vi "Producto extraccion.vi"(8 "error in (no error)":errorcluster, 10 "Indicador":dbl, 11 "Productos in":refnum<class "Productos.lvclass">) -> (0 "error out":errorcluster, 3 "Productos out":refnum<class "Productos.lvclass">)   [LabVIEW 2021, in "Productos.lvlib" / "Productos.lvclass"]
uses:
  Productos.lvclass
  Productos.lvclass/Productos.ctl
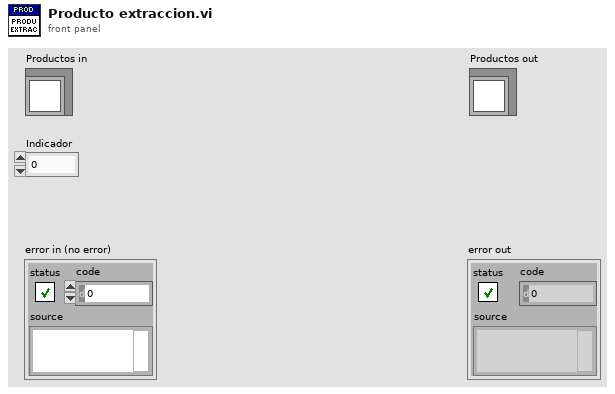
[diagram p1: front panel]
types:
  T1 = cluster{"Coca Cola":cluster{"Precio":dbl, "Stock":dbl}, "Pepsi":cluster{"Precio":dbl, "Stock":dbl}, "Doritos":cluster{"Precio":dbl, "Stock":dbl}, "Sabritas":cluster{"Precio":dbl, "Stock":dbl}, "Chocolate":cluster{"Precio":dbl, "Stock":dbl}, "Galletas":cluster{"Precio":dbl, "Stock":dbl}, "Cacahuates":cluster{"Precio":dbl, "Stock":dbl}, "Chicles":cluster{"Precio":dbl, "Stock":dbl}}
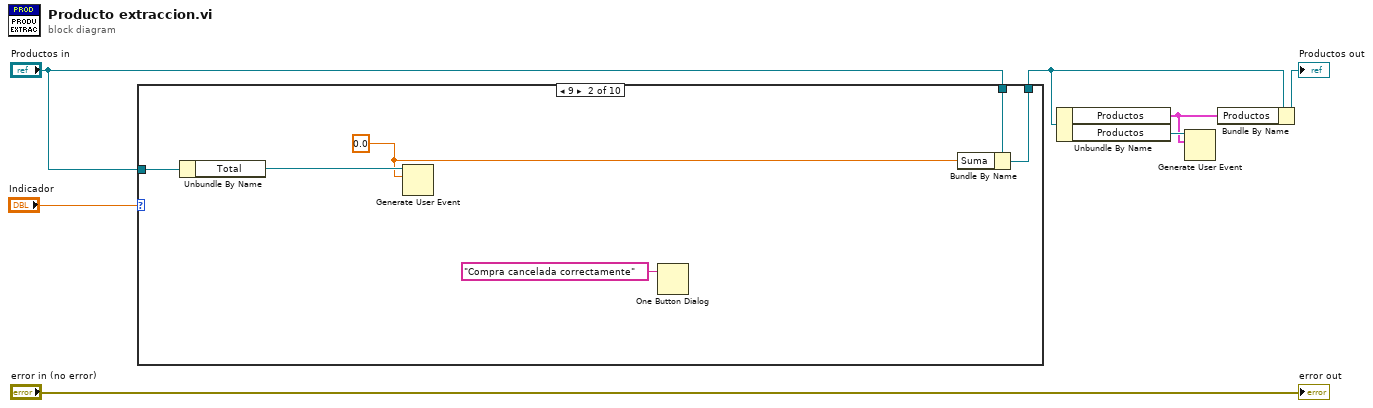
[diagram p0: block diagram]
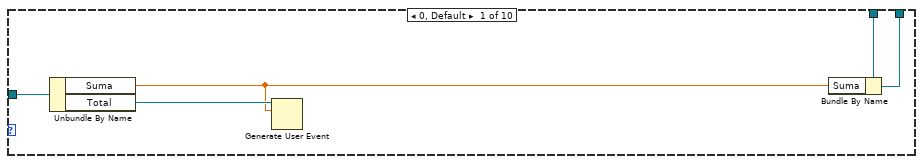
[diagram p2: hidden frame]
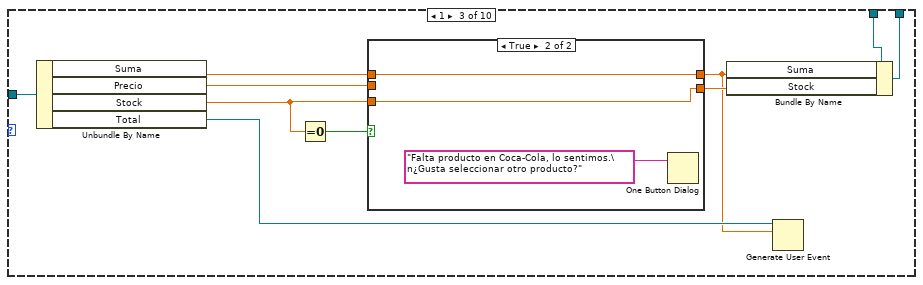
[diagram p3: hidden frame]
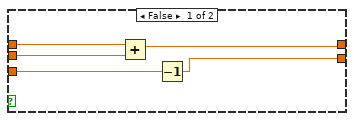
[diagram p4: hidden frame]
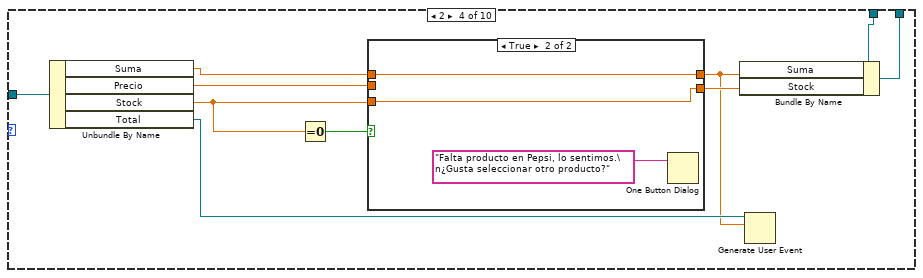
[diagram p5: hidden frame]
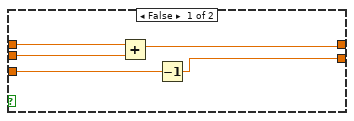
[diagram p6: hidden frame]
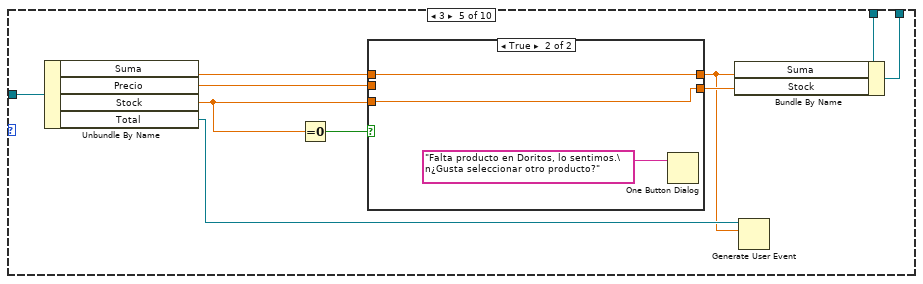
[diagram p7: hidden frame]
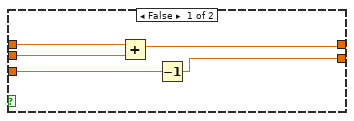
[diagram p8: hidden frame]
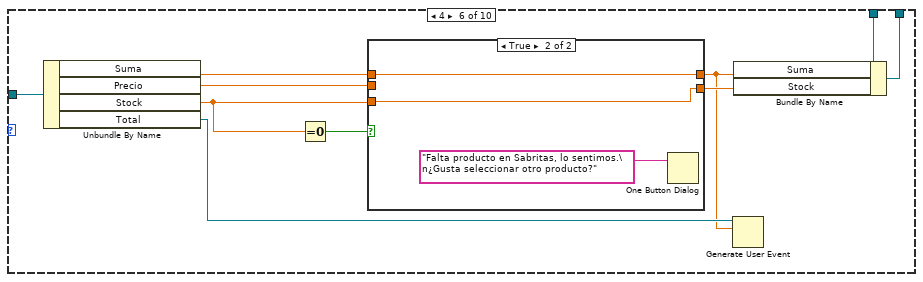
[diagram p9: hidden frame]
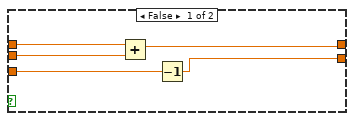
[diagram p10: hidden frame]
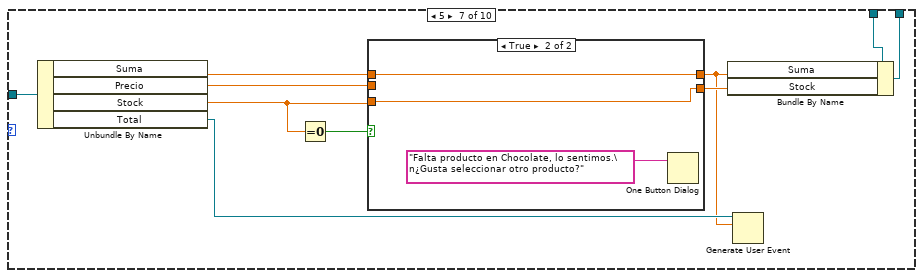
[diagram p11: hidden frame]
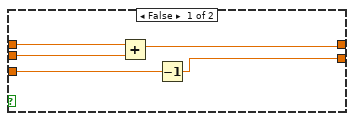
[diagram p12: hidden frame]
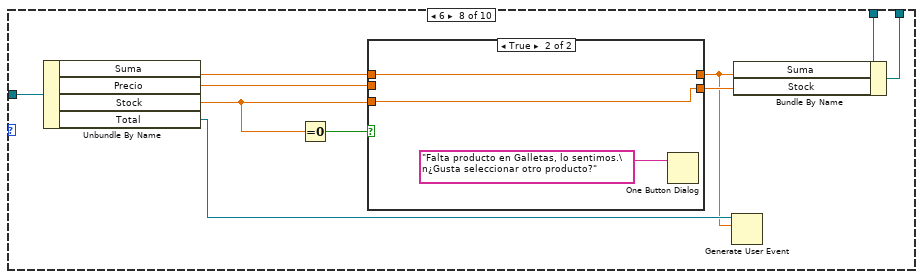
[diagram p13: hidden frame]
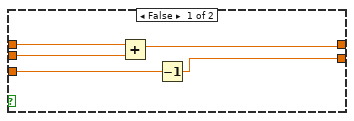
[diagram p14: hidden frame]
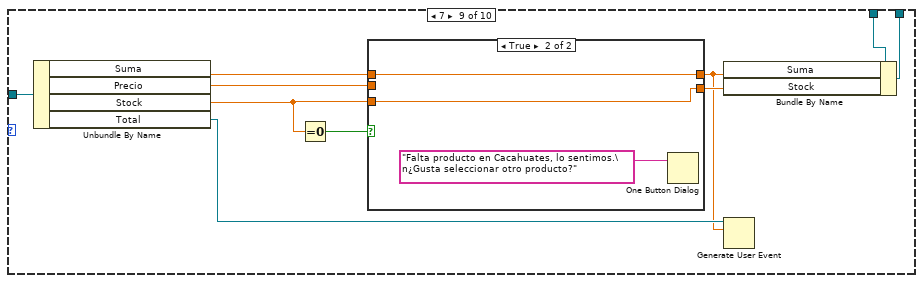
[diagram p15: hidden frame]
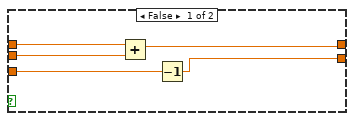
[diagram p16: hidden frame]
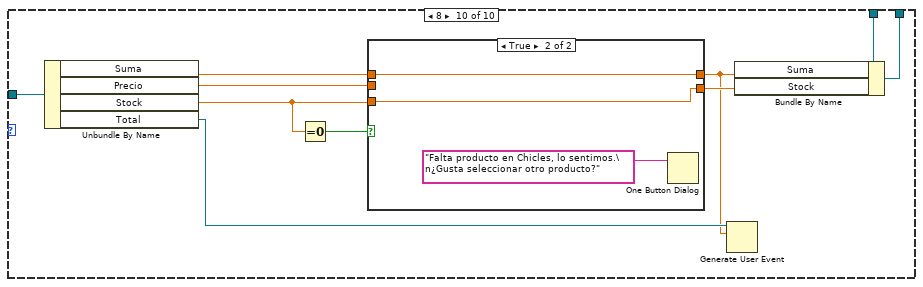
[diagram p17: hidden frame]
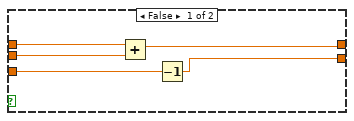
[diagram p18: hidden frame]
diagram:
  n1 = case shown="9" "Indicador" {
    tunnel: "Productos in" -> [w10 w16 w28 w46 w64 w82 w100 w118 w136 w154]
    tunnel: "Productos in" -> [w12 w18 w26 w44 w62 w80 w98 w116 w134 w152]
    tunnel: [w11 w17 w25 w42 w60 w78 w96 w114 w132 w150] -> w4
    frame 0, Default {
      n2 = Unbundle By Name(w10) -> ("Suma"=w8:dbl, "Total"=w9:refnum<user-event>)
      n3 = Generate User Event(user event=w9, event data cluster=w8) -> ()  [unwired: 2 in, 2 out]
      n4 = Bundle By Name(cluster=w12, "Suma"=w8) -> (w11:refnum<class "Productos.lvclass">)
    }
    frame 9 {
      w14 = 0.0 ("Suma")
      n5 = Unbundle By Name(w16) -> ("Total"=w15:refnum<user-event>)
      n6 = Generate User Event(user event=w15, event data cluster=w14) -> ()  [unwired: 2 in, 2 out]
      n7 = One Button Dialog(message="Compra cancelada correctamente") -> ()  [unwired: 1 in, 1 out]
      n8 = Bundle By Name(cluster=w18, "Suma"=w14) -> (w17:refnum<class "Productos.lvclass">)
    }
    frame 1 {
      n9 = Unbundle By Name(w28) -> ("Suma"=w20:dbl, "Precio"=w23:dbl, "Stock"=w22:dbl, "Total"=w21:refnum<user-event>)
      n10 = Equal To 0?(x=w22) -> (x = 0?=w27:bool)
      n11 = case shown="True" w27 {
        tunnel: w22 -> [w30 w34]
        tunnel: w23 -> [w33 _]
        tunnel: w20 -> [w32 w35]
        tunnel: [w31 w35] -> w19
        tunnel: [w29 w34] -> w24
        frame False {
          n12 = Add(x=w32, y=w33) -> (x+y=w31:dbl)
          n13 = Decrement(x=w30) -> (x-1=w29:dbl)
        }
        frame True {
          n14 = One Button Dialog(message="Falta producto en Coca-Cola, lo sentimos.\n¿Gusta seleccionar otro producto?") -> ()  [unwired: 1 in, 1 out]
        }
      }
      n15 = Bundle By Name(cluster=w26, "Suma"=w19, "Stock"=w24) -> (w25:refnum<class "Productos.lvclass">)
      n16 = Generate User Event(user event=w21, event data cluster=w19) -> ()  [unwired: 2 in, 2 out]
    }
    frame 2 {
      n17 = Unbundle By Name(w46) -> ("Suma"=w43:dbl, "Precio"=w40:dbl, "Stock"=w39:dbl, "Total"=w38:refnum<user-event>)
      n18 = Equal To 0?(x=w39) -> (x = 0?=w45:bool)
      n19 = case shown="True" w45 {
        tunnel: w39 -> [w48 w52]
        tunnel: w40 -> [w51 _]
        tunnel: w43 -> [w50 w53]
        tunnel: [w49 w53] -> w37
        tunnel: [w47 w52] -> w41
        frame False {
          n20 = Add(x=w50, y=w51) -> (x+y=w49:dbl)
          n21 = Decrement(x=w48) -> (x-1=w47:dbl)
        }
        frame True {
          n22 = One Button Dialog(message="Falta producto en Pepsi, lo sentimos.\n¿Gusta seleccionar otro producto?") -> ()  [unwired: 1 in, 1 out]
        }
      }
      n23 = Bundle By Name(cluster=w44, "Suma"=w37, "Stock"=w41) -> (w42:refnum<class "Productos.lvclass">)
      n24 = Generate User Event(user event=w38, event data cluster=w37) -> ()  [unwired: 2 in, 2 out]
    }
    frame 3 {
      n25 = Unbundle By Name(w64) -> ("Suma"=w61:dbl, "Precio"=w58:dbl, "Stock"=w57:dbl, "Total"=w56:refnum<user-event>)
      n26 = Equal To 0?(x=w57) -> (x = 0?=w63:bool)
      n27 = case shown="True" w63 {
        tunnel: w57 -> [w66 w70]
        tunnel: w58 -> [w69 _]
        tunnel: w61 -> [w68 w71]
        tunnel: [w67 w71] -> w55
        tunnel: [w65 w70] -> w59
        frame False {
          n28 = Add(x=w68, y=w69) -> (x+y=w67:dbl)
          n29 = Decrement(x=w66) -> (x-1=w65:dbl)
        }
        frame True {
          n30 = One Button Dialog(message="Falta producto en Doritos, lo sentimos.\n¿Gusta seleccionar otro producto?") -> ()  [unwired: 1 in, 1 out]
        }
      }
      n31 = Bundle By Name(cluster=w62, "Suma"=w55, "Stock"=w59) -> (w60:refnum<class "Productos.lvclass">)
      n32 = Generate User Event(user event=w56, event data cluster=w55) -> ()  [unwired: 2 in, 2 out]
    }
    frame 4 {
      n33 = Unbundle By Name(w82) -> ("Suma"=w79:dbl, "Precio"=w76:dbl, "Stock"=w75:dbl, "Total"=w74:refnum<user-event>)
      n34 = Equal To 0?(x=w75) -> (x = 0?=w81:bool)
      n35 = case shown="True" w81 {
        tunnel: w75 -> [w84 w88]
        tunnel: w76 -> [w87 _]
        tunnel: w79 -> [w86 w89]
        tunnel: [w85 w89] -> w73
        tunnel: [w83 w88] -> w77
        frame False {
          n36 = Add(x=w86, y=w87) -> (x+y=w85:dbl)
          n37 = Decrement(x=w84) -> (x-1=w83:dbl)
        }
        frame True {
          n38 = One Button Dialog(message="Falta producto en Sabritas, lo sentimos.\n¿Gusta seleccionar otro producto?") -> ()  [unwired: 1 in, 1 out]
        }
      }
      n39 = Generate User Event(user event=w74, event data cluster=w73) -> ()  [unwired: 2 in, 2 out]
      n40 = Bundle By Name(cluster=w80, "Suma"=w73, "Stock"=w77) -> (w78:refnum<class "Productos.lvclass">)
    }
    frame 5 {
      n41 = Unbundle By Name(w100) -> ("Suma"=w97:dbl, "Precio"=w94:dbl, "Stock"=w93:dbl, "Total"=w92:refnum<user-event>)
      n42 = Equal To 0?(x=w93) -> (x = 0?=w99:bool)
      n43 = case shown="True" w99 {
        tunnel: w93 -> [w102 w106]
        tunnel: w94 -> [w105 _]
        tunnel: w97 -> [w104 w107]
        tunnel: [w103 w107] -> w91
        tunnel: [w101 w106] -> w95
        frame False {
          n44 = Add(x=w104, y=w105) -> (x+y=w103:dbl)
          n45 = Decrement(x=w102) -> (x-1=w101:dbl)
        }
        frame True {
          n46 = One Button Dialog(message="Falta producto en Chocolate, lo sentimos.\n¿Gusta seleccionar otro producto?") -> ()  [unwired: 1 in, 1 out]
        }
      }
      n47 = Bundle By Name(cluster=w98, "Suma"=w91, "Stock"=w95) -> (w96:refnum<class "Productos.lvclass">)
      n48 = Generate User Event(user event=w92, event data cluster=w91) -> ()  [unwired: 2 in, 2 out]
    }
    frame 6 {
      n49 = Unbundle By Name(w118) -> ("Suma"=w115:dbl, "Precio"=w112:dbl, "Stock"=w111:dbl, "Total"=w110:refnum<user-event>)
      n50 = Equal To 0?(x=w111) -> (x = 0?=w117:bool)
      n51 = case shown="True" w117 {
        tunnel: w111 -> [w120 w124]
        tunnel: w112 -> [w123 _]
        tunnel: w115 -> [w122 w125]
        tunnel: [w121 w125] -> w109
        tunnel: [w119 w124] -> w113
        frame False {
          n52 = Add(x=w122, y=w123) -> (x+y=w121:dbl)
          n53 = Decrement(x=w120) -> (x-1=w119:dbl)
        }
        frame True {
          n54 = One Button Dialog(message="Falta producto en Galletas, lo sentimos.\n¿Gusta seleccionar otro producto?") -> ()  [unwired: 1 in, 1 out]
        }
      }
      n55 = Generate User Event(user event=w110, event data cluster=w109) -> ()  [unwired: 2 in, 2 out]
      n56 = Bundle By Name(cluster=w116, "Suma"=w109, "Stock"=w113) -> (w114:refnum<class "Productos.lvclass">)
    }
    frame 7 {
      n57 = Unbundle By Name(w136) -> ("Suma"=w133:dbl, "Precio"=w130:dbl, "Stock"=w129:dbl, "Total"=w128:refnum<user-event>)
      n58 = Equal To 0?(x=w129) -> (x = 0?=w135:bool)
      n59 = case shown="True" w135 {
        tunnel: w129 -> [w138 w142]
        tunnel: w130 -> [w141 _]
        tunnel: w133 -> [w140 w143]
        tunnel: [w139 w143] -> w127
        tunnel: [w137 w142] -> w131
        frame False {
          n60 = Add(x=w140, y=w141) -> (x+y=w139:dbl)
          n61 = Decrement(x=w138) -> (x-1=w137:dbl)
        }
        frame True {
          n62 = One Button Dialog(message="Falta producto en Cacahuates, lo sentimos.\n¿Gusta seleccionar otro producto?") -> ()  [unwired: 1 in, 1 out]
        }
      }
      n63 = Bundle By Name(cluster=w134, "Suma"=w127, "Stock"=w131) -> (w132:refnum<class "Productos.lvclass">)
      n64 = Generate User Event(user event=w128, event data cluster=w127) -> ()  [unwired: 2 in, 2 out]
    }
    frame 8 {
      n65 = Unbundle By Name(w154) -> ("Suma"=w151:dbl, "Precio"=w148:dbl, "Stock"=w147:dbl, "Total"=w146:refnum<user-event>)
      n66 = Equal To 0?(x=w147) -> (x = 0?=w153:bool)
      n67 = case shown="True" w153 {
        tunnel: w147 -> [w156 w160]
        tunnel: w148 -> [w159 _]
        tunnel: w151 -> [w158 w161]
        tunnel: [w157 w161] -> w145
        tunnel: [w155 w160] -> w149
        frame False {
          n68 = Add(x=w158, y=w159) -> (x+y=w157:dbl)
          n69 = Decrement(x=w156) -> (x-1=w155:dbl)
        }
        frame True {
          n70 = One Button Dialog(message="Falta producto en Chicles, lo sentimos.\n¿Gusta seleccionar otro producto?") -> ()  [unwired: 1 in, 1 out]
        }
      }
      n71 = Generate User Event(user event=w146, event data cluster=w145) -> ()  [unwired: 2 in, 2 out]
      n72 = Bundle By Name(cluster=w152, "Suma"=w145, "Stock"=w149) -> (w150:refnum<class "Productos.lvclass">)
    }
  }
  n73 = Unbundle By Name(w4) -> ("Productos"=w1:T1, "Productos"=w3:refnum<user-event>)
  n74 = Generate User Event(user event=w3, event data cluster=w1) -> ()  [unwired: 2 in, 2 out]
  n75 = Bundle By Name(cluster=w4, "Productos"=w1) -> (→"Productos out":refnum<class "Productos.lvclass">)
  "error out" <- "error in (no error)"
